vi "oa_Get FIR Filter Length.vi"(7 "reset? (T)":bool=TRUE, 8 "FIR filter specifications":T1={"alias rejection (dB)"=125.0, "normalized bandwidth"=0.4536} {"normalized bandwidth" format="%.4f"; "alias rejection (dB)" format="%.2f"}, 10 "dr new":dbl=1.0 format="%.2p", 11 "dr old":dbl=1.0 format="%.2p") -> (1 "filter length":i32, 2 "dr old out":dbl=1.0 format="%.2p")   [LabVIEW 2017, in "SoundVib_OAUtility.lvlib"]
uses:
  <vilib>/addons/Sound and Vibration/Order Analysis/Utility/SoundVib_OAUtility.lvlib
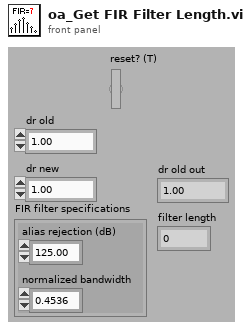
[diagram p1: front panel]
types:
  T1 = cluster{"alias rejection (dB)":dbl, "normalized bandwidth":dbl}
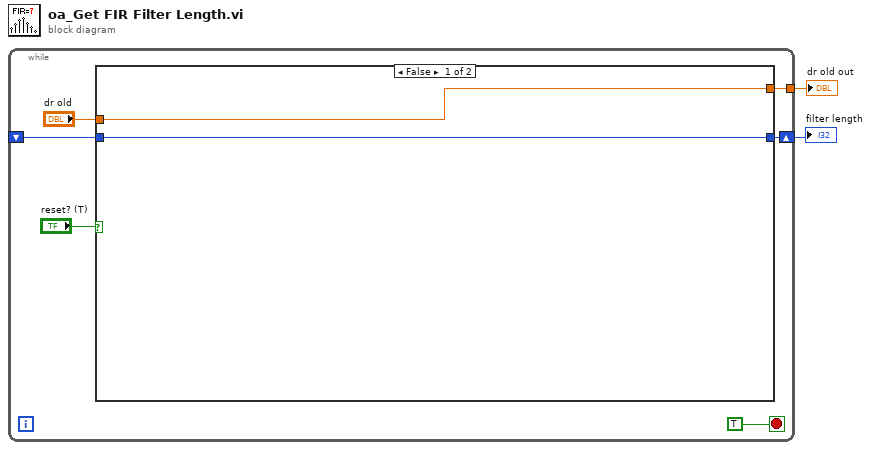
[diagram p0: block diagram]
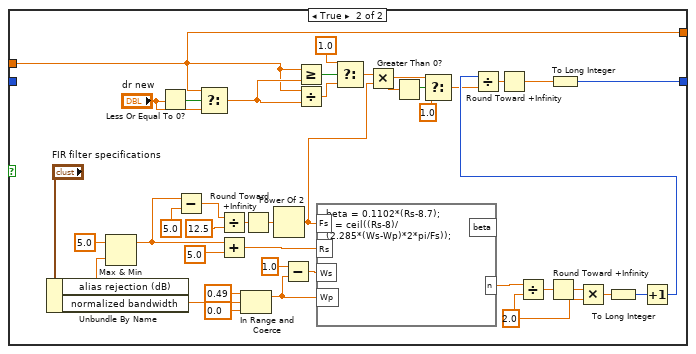
[diagram p2: hidden frame]
diagram:
  n1 = while {
    shift-right: [w6] -> w2
    shift-left: _ -> [w5]
    tunnel: [w3] -> w1
    stop <- TRUE stop-if-true
    n2 = case shown="False" "reset? (T)" {
      tunnel: [w10 w12] -> w6
      tunnel: w5 -> [w10 _]
      tunnel: "dr old" -> [w9 w11]
      tunnel: [w9 w11] -> w3
      frame False {
      }
      frame True {
        w46 = 2.0 ("y")
        n3 = Unbundle By Name("FIR filter specifications") -> ("alias rejection (dB)"=w30:dbl, "normalized bandwidth"=w34:dbl)
        n4 = Max & Min(x=5.0, y=w30) -> (max(x,y)=w31:dbl)  [unwired: 1 out]
        n5 = Less Or Equal To 0?(x="dr new") -> (x <= 0?=w20:bool)
        n6 = Subtract(x=w31, y=5.0) -> (x-y=w40:dbl)
        n7 = Select(t=w11, s=w20, f="dr new") -> (s? t:f=w18:dbl)
        n8 = Divide(x=w40, y=12.5) -> (x/y=w39:dbl)
        n9 = Add(x=w31, y=5.0) -> (x+y=w38:dbl)
        n10 = In Range and Coerce(upper limit=0.49, x=w34, lower limit=0.0) -> (coerced(x)=w35:dbl)  [unwired: 1 out]
        n11 = Round Toward +Infinity(x=w39) -> (ceil(x): smallest int >= x=w43:dbl)
        n12 = Power Of 2(x=w43) -> (2^x=w21:dbl)
        n13 = Subtract(x=1.0, y=w35) -> (x-y=w44:dbl)
        n14 = Greater Or Equal?(x=w11, y=w18) -> (x >= y?=w27:bool)
        n15 = Divide(x=w11, y=w18) -> (x/y=w25:dbl)
        n16 = formula code="beta = 0.1102*(Rs-8.7);\nn = ceil((Rs-8)/(2.285*(Ws-Wp)*2*pi/Fs));"("Rs"=w38, "Ws"=w44, "Wp"=w35, "Fs"=w21) -> ("n"=w50:dbl)  [unwired: 1 out]
        n17 = Select(t=1.0, s=w27, f=w25) -> (s? t:f=w24:dbl)
        n18 = Multiply(x=w24, y=w21) -> (x*y=w16:dbl)
        n19 = Greater Than 0?(x=w16) -> (x > 0?=w17:bool)
        n20 = Select(t=w16, s=w17, f=1.0) -> (s? t:f=w14:dbl)
        n21 = Divide(x=w50, y=w46) -> (x/y=w48:dbl)
        n22 = Round Toward +Infinity(x=w48) -> (ceil(x): smallest int >= x=w47:dbl)
        n23 = Multiply(x=w47, y=w46) -> (x*y=w49:dbl)
        n24 = To Long Integer(number=w49) -> (32bit integer=w28:i32)
        n25 = Increment(x=w28) -> (x+1=w23:i32)
        n26 = Divide(x=w23, y=w14) -> (x/y=w22:dbl)
        n27 = Round Toward +Infinity(x=w22) -> (ceil(x): smallest int >= x=w13:dbl)
        n28 = To Long Integer(number=w13) -> (32bit integer=w12:i32)
      }
    }
  }
  "filter length" <- w2
  "dr old out" <- w1
